vi "Configure Marker State.vi"(7 "Maker On (F)":bool, 8 "error in (no error)":errorcluster, 10 "Marker Number (1)":u32=1 min=1, 11 "SA-FSW in":refnum<class "SA-FSW.lvclass">) -> (0 "error out":errorcluster, 3 "SA-FSW out":refnum<class "SA-FSW.lvclass">)   [LabVIEW 2020, in "SA-FSW.lvclass"]
uses:
  SA-FSW.lvclass
  C:/Sandbox/RF Bench/Source Code/WiSpry Test Framework/Instruments/Instrument.lvclass
  Instrument.lvclass/Instrument.ctl
  Instrument.lvclass
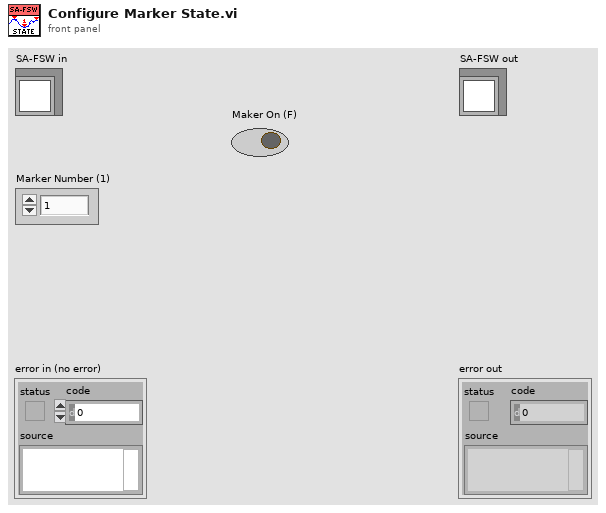
[diagram p1: front panel]
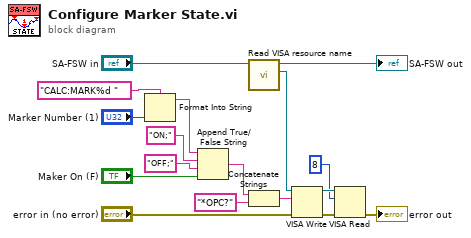
[diagram p0: block diagram]
diagram:
  n1 = Format Into String(format string="CALC:MARK%d ", "Marker Number (1)") -> (resulting string=w15:string)  [unwired: 2 in, 1 out]
  n2 = Append True/False String(1:"Maker On (F)", 2:"OFF;" ("false string"), 3:"ON;" ("true string"), 4:w15) -> (0:w11:string)
  n3 = call "Read VISA resource name.vi"("Instrument in"="SA-FSW in") -> ("VISA resource name"=w7:refnum<visa-resource-name>, "Instrument out"=→"SA-FSW out":refnum<class "SA-FSW.lvclass">)  [unwired: 9 in]
  n4 = Concatenate Strings(w11, "*OPC?" ("string")) -> (w8:string)
  n5 = VISA Write(VISA resource name=w7, write buffer=w8, error in (no error)="error in (no error)") -> (VISA resource name out=w5:refnum<visa-resource-name>, error out=w4:errorcluster)  [unwired: 1 out]
  n6 = VISA Read(VISA resource name=w5, byte count=u32 8, error in (no error)=w4) -> (error out=→"error out":errorcluster)  [unwired: 3 out]
